vi "robotFriction.vi"(8 "V in":dbl, 9 "F in":dbl, 10 "coeff friction":dbl, 11 "Mass":dbl) -> (3 "Force out":dbl)   [LabVIEW 2017]
panel:
  out "Friction":dbl
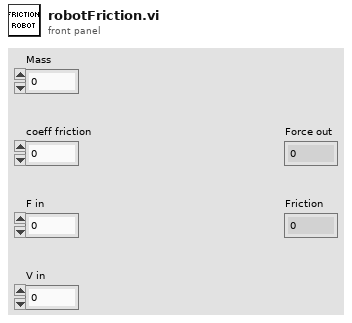
[diagram p1: front panel]
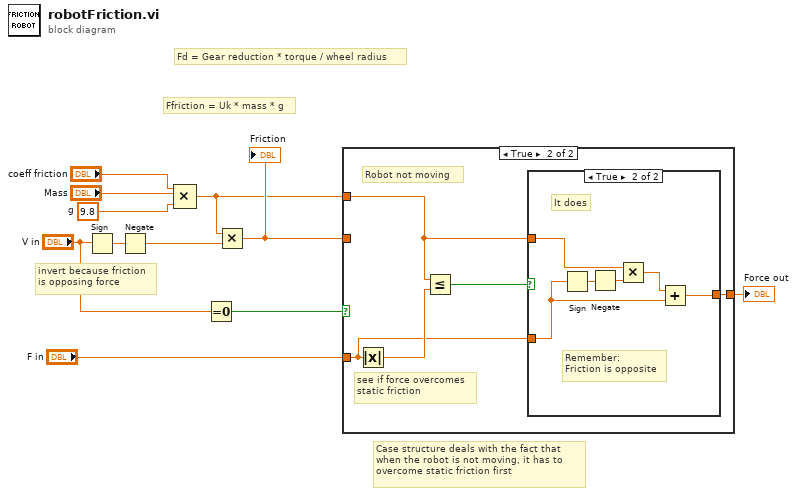
[diagram p0: block diagram]
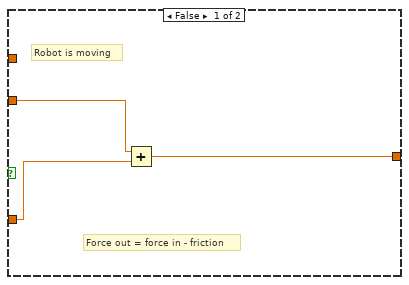
[diagram p2: hidden frame]
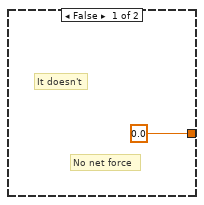
[diagram p3: hidden frame]
diagram:
  w9 = 9.8  # g
  # "Case structure deals with the fact that\nwhen the robot is not moving, it has to \novercome static friction first"
  # "invert because friction\nis opposing force"
  # "Ffriction = Uk * mass * g"
  # "Fd = Gear reduction * torque / wheel radius"
  n1 = Sign(1:"V in") -> (0:w8:dbl)
  n2 = Negate(x=w8) -> (-x=w7:dbl)
  n3 = Compound Arithmetic op=MULTIPLY("coeff friction", "Mass", w9) -> (w5:dbl)
  n4 = Equal To 0?(x="V in") -> (x = 0?=w2:bool)
  n5 = Multiply(x=w5, y=w7) -> (x*y=w6:dbl)
  "Friction" <- w6
  n6 = case shown="True" w2 {
    tunnel: w6 -> [w14 _]
    tunnel: w5 -> [_ w15]
    tunnel: "F in" -> [w13 w17]
    tunnel: [w12 w16] -> w1
    frame False {
      # "Force out = force in - friction"
      # "Robot is moving"
      n7 = Add(x=w14, y=w13) -> (x+y=w12:dbl)
    }
    frame True {
      # "see if force overcomes\nstatic friction"
      # "Robot not moving"
      n8 = Absolute Value(x=w17) -> (abs(x)=w18:dbl)
      n9 = Less Or Equal?(x=w15, y=w18) -> (x <= y?=w19:bool)
      n10 = case shown="True" w19 {
        tunnel: w17 -> [_ w25]
        tunnel: [0.0 ("F in") w26] -> w16
        tunnel: w15 -> [_ w24]
        frame False {
          # "No net force"
          # "It doesn't"
        }
        frame True {
          # "Remember:\nFriction is opposite"
          # "It does"
          n11 = Sign(1:w25) -> (0:w23:dbl)
          n12 = Negate(x=w23) -> (-x=w22:dbl)
          n13 = Multiply(x=w24, y=w22) -> (x*y=w21:dbl)
          n14 = Add(x=w21, y=w25) -> (x+y=w26:dbl)
        }
      }
    }
  }
  "Force out" <- w1
